vi "M227_Quit.vi"(11 "VISA Refnum in":refnum<visa-resource-name>) -> ()   [LabVIEW 2011]
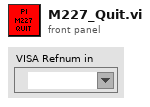
[diagram p1: front panel]
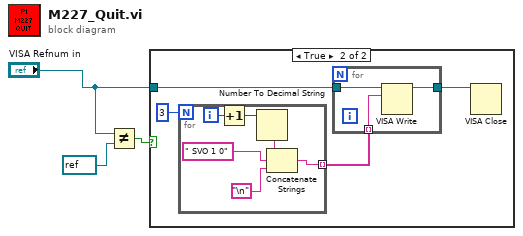
[diagram p0: block diagram]
diagram:
  n1 = Not Equal?(x="VISA Refnum in", y=refnum<visa-resource-name> refnum ("VISA resource name")) -> (x != y?=w1:bool)
  n2 = case shown="True" w1 {
    tunnel: "VISA Refnum in" -> [_ w7]
    frame False {
    }
    frame True {
      n3 = for {
        N: 3 -> [_]
        tunnel: [w13] -> w4 mode=indexing
        i -> [w11]
        n4 = Increment(x=w11) -> (x+1=w12:i32)
        n5 = Number To Decimal String(number=w12) -> (decimal integer string=w9:string)  [unwired: 1 in]
        n6 = Concatenate Strings(w9, " SVO 1 0" ("string"), "\n") -> (w13:string)
      }
      n7 = for {
        tunnel: w7 -> [w16]
        tunnel: [w15] -> w5
        tunnel: w4 -> [w14] mode=indexing
        n8 = VISA Write(VISA resource name=w16, write buffer=w14) -> (VISA resource name out=w15:refnum<visa-resource-name>)  [unwired: 1 in, 2 out]
      }
      n9 = VISA Close(VISA resource name=w5) -> ()  [unwired: 1 in, 1 out]
    }
  }
